vi "From Serial Form.vi"(6 "Serial Version":T1, 10 "Deserializer in":refnum<class "Deserializer.lvclass">, 11 "BrowerLeaf in":refnum<class "BrowerLeaf.lvclass">) -> (0 "error out":errorcluster, 2 "Deserializer out":refnum<class "Deserializer.lvclass">, 3 "BrowerLeaf out":refnum<class "BrowerLeaf.lvclass">)   [LabVIEW 2015, in "BrowerLeaf.lvclass"]
uses:
  BrowerLeaf.lvclass
  <vilib>/NI/AQ Character Lineator/Deserializer/Deserializer.lvclass
  <vilib>/NI/AQ Character Lineator/Serialization Common/Serial Version.ctl
  BrowerComponent/BrowerComponent.lvclass
  <vilib>/NI/AQ Character Lineator/Serialization Common/Serialization Common.lvlib
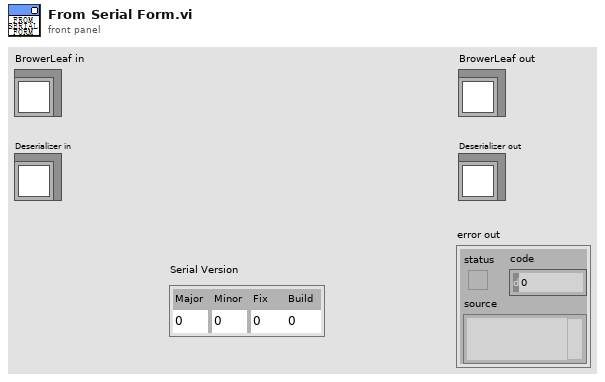
[diagram p1: front panel]
types:
  T1 = typedef "Serialization Common.lvlib/Serial Version.ctl" = cluster{"Major":u16, "Minor":u16, "Fix":u16, "Build":u16}
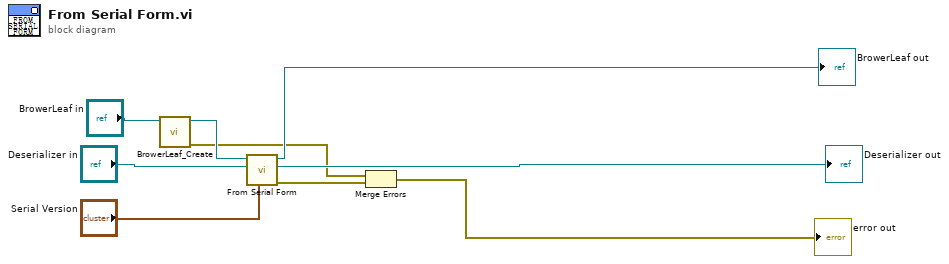
[diagram p0: block diagram]
diagram:
  n1 = call "BrowerLeaf_Create.vi"("reference in"="BrowerLeaf in") -> ("error out"=w3:errorcluster, "reference out"=w5:refnum<class "BrowerLeaf.lvclass">)  [unwired: 9 in]
  n2 = call-parent "From Serial Form.vi"("Serial Version"="Serial Version", "Deserializer in"="Deserializer in", "BrowerComponent in"=w5) -> ("error out"=w2:errorcluster, "Deserializer out"=→"Deserializer out":refnum<class "Deserializer.lvclass">, "BrowerComponent out"=→"BrowerLeaf out":refnum<class "BrowerLeaf.lvclass">)  [unwired: 6 in]
  n3 = Merge Errors(w3, w2) -> (→"error out":errorcluster)
